vi "Function_Flow Mark #2.vi"(8 "Error in":errorcluster, 9 "CoordSys In":T2 {"Measurement System"."Axis Reference" items=["Direct", "Indirect"]; "Measurement System"."Angle (deg)" format="%.2f"; "Measurement System"."Origin"."Y" format="%.2f"; "Measurement System"."Origin"."X" format="%.2f"; "Reference System"."Axis Reference" items=["Direct", "Indirect"]; "Reference System"."Angle (deg)" format="%.2f"; "Reference System"."Origin"."Y" format="%.2f"; "Reference System"."Origin"."X" format="%.2f"}, 10 "Data Cluster In":cluster{"Name":string, "Variant In":variant}, 11 "Image Dst In":T4) -> (0 "Error out":errorcluster, 2 "ROI Descriptor out":T3 {"Contours"."Type" items=["No Selection", "Point", "Line", "Rectangle", "Oval", "Polygon", "Freehand Region", "Annulus", "Unused2", "Unused3", "Broken Line", "Freehand Line", "Rotated Rectangle"]}, 3 "Objects":T1(array[cluster]) {"Area" format="%.2f"; "Object Center"."Y" format="%.2f"; "Object Center"."X" format="%.2f"})   [LabVIEW 2013]
uses:
  <vilib>/vision/Image Controls.llb/IMAQ Image.ctl
  Control/Control_Flow Mark.ctl
  <vilib>/vision/NI_Vision_Development_Module.lvlib
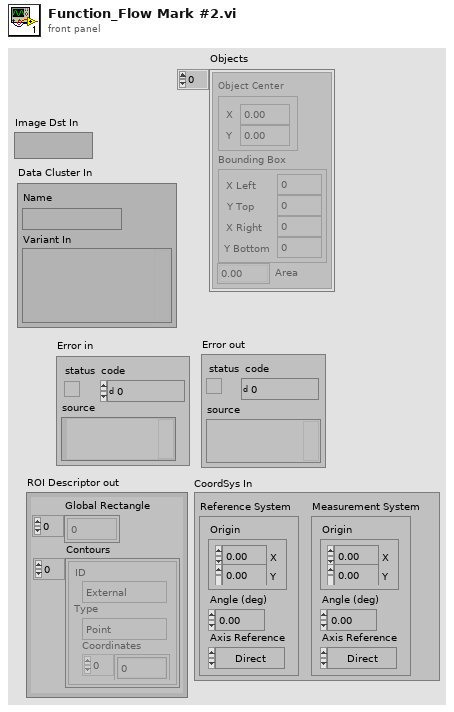
[diagram p1: front panel]
types:
  T1 = cluster{"Object Center":cluster{"X":dbl, "Y":dbl}, "Bounding Box":cluster{"X Left":dbl, "Y Top":dbl, "X Right":dbl, "Y Bottom":dbl}, "Area":dbl}[]
  T2 = typedef "IMAQ Coordinate System" = cluster{"Reference System":cluster{"Origin":cluster{"X":sgl, "Y":sgl}, "Angle (deg)":sgl, "Axis Reference":u32}, "Measurement System":cluster{"Origin":cluster{"X":sgl, "Y":sgl}, "Angle (deg)":sgl, "Axis Reference":u32}}
  T3 = typedef "ROI Descriptor" = cluster{"Global Rectangle":i32[], "Contours":cluster{"ID":enum32{"External", "Internal"}, "Type":u32, "Coordinates":i32[]}[]}
  T4 = typedef "IMAQ Image.ctl" = refnum<image>
  T5 = typedef "Control_Flow Mark.ctl" = cluster{"Name":string, "ROI":cluster{"Global Rectangle":i32[], "Contours":cluster{"ID":enum32{"External", "Internal"}, "Type":u32, "Coordinates":i32[]}[]}, "Extract Direction(¬y²ª)":enum16{"Left up", "Right up", "Left Down", "Right Down"}, "Extract Potion(¬y²ª)":cluster{"X":i32, "Y":i32}, "Magnification(¬y²ª)":i32, "Settings(¬y²ª)":cluster{"Objects":enum16{"Bright Objects", "Dark Objects"}, "Threshold":i32, "Min Object Size":bool, "Min Size":i32, "Max Object Size":bool, "Max Size":i32}}
  T6 = cluster{"Origin":cluster{"X":sgl, "Y":sgl}, "Angle (deg)":sgl, "Axis Reference":u32}
  T7 = cluster{"Global Rectangle":i32[], "Contours":cluster{"ID":enum32{"External", "Internal"}, "Type":u32, "Coordinates":i32[]}[]}
  T8 = enum16{"Left up", "Right up", "Left Down", "Right Down"}
  T9 = cluster{"Objects":enum16{"Bright Objects", "Dark Objects"}, "Threshold":i32, "Min Object Size":bool, "Min Size":i32, "Max Object Size":bool, "Max Size":i32}
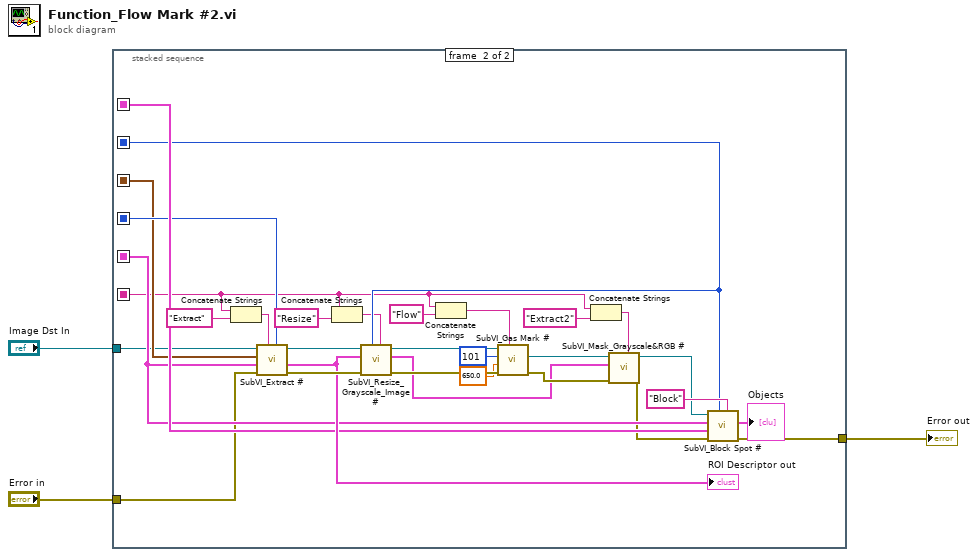
[diagram p0: block diagram]
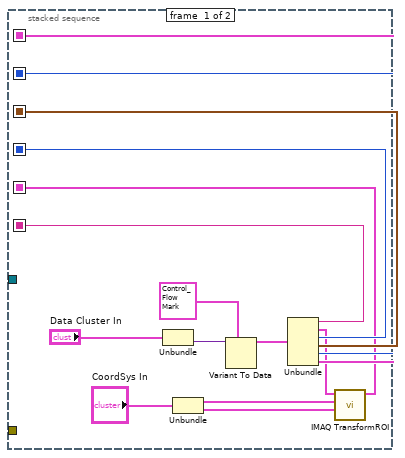
[diagram p2: hidden frame]
diagram:
  n1 = stacked-sequence {
    seq-local: [w14 _] -> [_ w20]
    seq-local: [w4 _] -> [_ w35]
    seq-local: [w13 _] -> [_ w33]
    seq-local: [w12 _] -> [_ w32]
    seq-local: [w11 _] -> [_ w34]
    seq-local: [w10 _] -> [_ w36]
    tunnel: "Image Dst In" -> [_ w31]
    tunnel: "Error in" -> [_ w30]
    tunnel: [_ w19] -> w1
    frame #0 {
      n2 = Unbundle("Data Cluster In") -> ("Variant In"=w16:variant)  [unwired: 1 out]
      n3 = Unbundle("CoordSys In") -> ("Reference System"=w7:T6, "Measurement System"=w6:T6)
      n4 = Variant To Data(type=T5 {"Name"="", "ROI"={"Global Rectangle"=[], "Contours"=[]}, "Extract Direction(¬y²ª)"=enum."Left up", "Extract Potion(¬y²ª)"={"X"=0, "Y"=0}, "Magnification(¬y²ª)"=2, "Settings(¬y²ª)"={"Objects"=enum."Dark Objects", "Threshold"=100, "Min Object Size"=TRUE, "Min Size"=6, "Max Object Size"=FALSE, "Max Size"=100}} ("¬y²ª_Setting"), Variant=w16) -> (data=w15:T5)  [unwired: 1 in, 1 out]
      n5 = Unbundle(w15) -> ("Name"=w14:string, "ROI"=w5:T7, "Extract Direction(¬y²ª)"=w13:T8, "Extract Potion(¬y²ª)"=w12:cluster{"X":i32, "Y":i32}, "Magnification(¬y²ª)"=w11:i32, "Settings(¬y²ª)"=w10:T9)
      n6 = call "IMAQ TransformROI"("New Reference"=w6, "Base Reference"=w7, "ROI Descriptor"=w5) -> ("ROI Descriptor out"=w4:T3)  [unwired: 7 in, 1 out]
    }
    frame #1 {
      n7 = Concatenate Strings(w20, "Extract" ("Image Register Name")) -> (w27:string)
      n8 = call "SubVI_Extract #.vi"("Extract Direction"=w33, "Image Register Name"=w27, "Error in"=w30, "ROI Descriptor"=w35, "Extract Potion"=w32, "Image In"=w31) -> ("Error out"=w46:errorcluster, "ROI Descriptor out"=w38:T3, "Image Dst Out"=w39:T4)  [unwired: 3 in]
      "ROI Descriptor out" <- w38
      n9 = Concatenate Strings(w20, "Resize" ("Image Register Name")) -> (w25:string)
      n10 = call "SubVI_Resize_Grayscale_Image #.vi"("Image Register Name"=w25, "Magnification"=w34, "Error In"=w46, "ROI Descriptor"=w38, "Image In"=w39) -> ("Error Out"=w47:errorcluster, "ROI Descriptor out"=w37:T3, "Image Out"=w40:T4)  [unwired: 4 in]
      n11 = Concatenate Strings(w20, "Flow" ("Image Register Name")) -> (w24:string)
      n12 = call "SubVI_Gas Mark #.vi"("Image Register Name"=w24, "Error in"=w47, "Divider"=sgl 650.0, "Kernel Size"=101, "Image Src In"=w40) -> ("Error out"=w48:errorcluster, "Image Dst Out"=w41:T4)  [unwired: 4 in, 1 out]
      n13 = Concatenate Strings(w20, "Extract2" ("Image Register Name")) -> (w21:string)
      n14 = call "SubVI_Mask_Grayscale&RGB #.vi"("Image Register Name"=w21, "Error in"=w48, "ROI Descriptor"=w37, "Image Src In"=w41) -> ("Error out"=w29:errorcluster, "Image Dst Out"=w42:T4)  [unwired: 5 in, 1 out]
      n15 = call "SubVI_Block Spot #.vi"("Image Register Name"="Block", "Magnification"=w34, "Error in"=w29, "Settings"=w36, "ROI Descriptor"=w35, "Image In"=w42) -> ("Error out"=w19:errorcluster, "Objects"=→"Objects":T1)  [unwired: 4 in]
    }
  }
  "Error out" <- w1
